vi "Test Save Unicode Paths.vi"(8 "error in (no error)":errorcluster) -> (0 "error out":errorcluster, 3 "Pass?":bool)   [LabVIEW 2020]
uses:
  <vilib>/picture/picture.llb/imagedata.ctl
  G-Image/Image IO/Polymorphic VIs/Save BMP Image (UTF-8 Path).vi
  G-Image/Image IO/Polymorphic VIs/Save GIF Image (UTF-8 Path).vi
  G-Image/Image IO/Polymorphic VIs/Save JPG Image (UTF-8 Path).vi
  G-Image/Image IO/Polymorphic VIs/Save PNG Image (UTF-8 Path).vi
  G-Image/Image IO/Polymorphic VIs/Save QOI Image (UTF-8 Path).vi
  G-Image/Image IO/Polymorphic VIs/Save TGA Image (UTF-8 Path).vi
  G-Image/Image IO/Polymorphic VIs/Load Image (UTF-8 Path).vi
  G-Image/G-Image.lvlib
panel:
  out "Array":cluster{string, "new picture":picture}[](array[cluster])
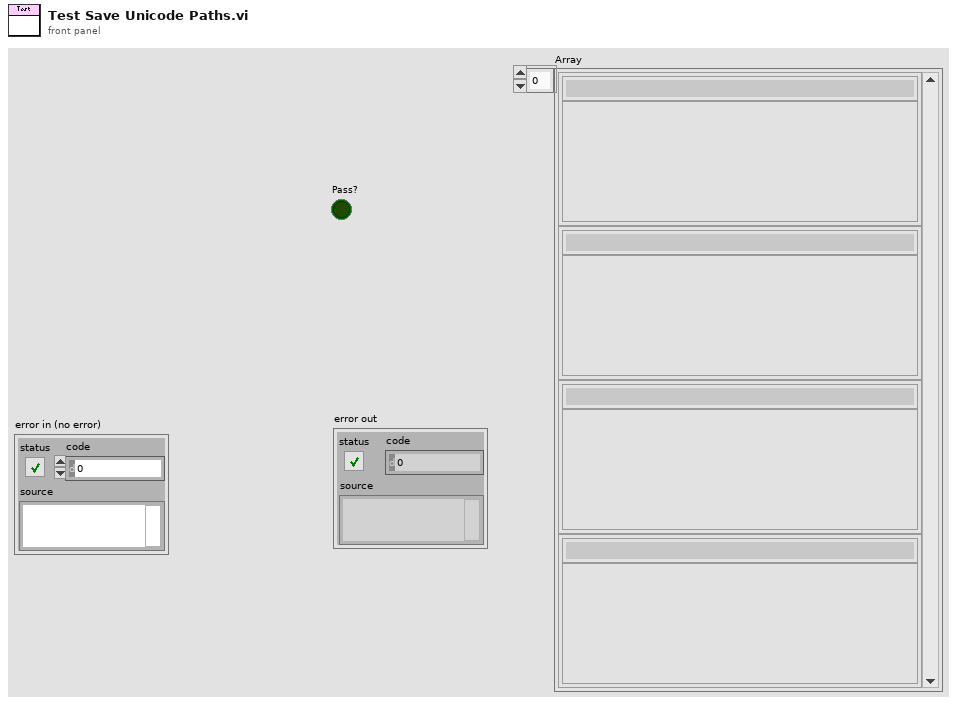
[diagram p1: front panel]
types:
  T1 = typedef "imagedata.ctl" = cluster{"image type":i32, "image depth":i32, "image":u8[], "mask":u8[], "colors":u32[], "Rectangle":cluster{"left":i16, "top":i16, "right":i16, "bottom":i16}}
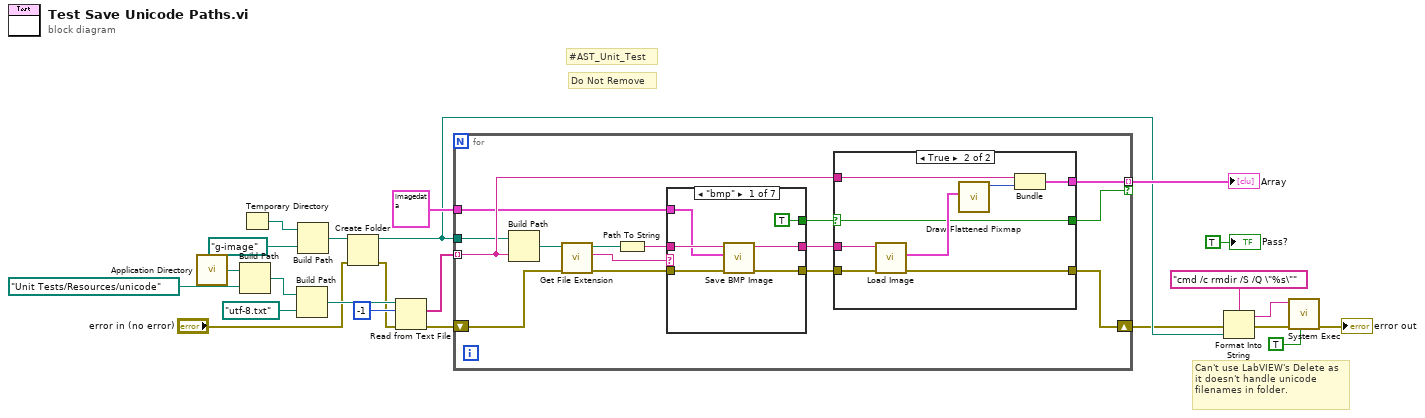
[diagram p0: block diagram]
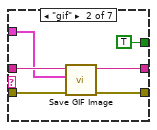
[diagram p3: hidden frame]
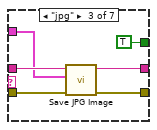
[diagram p4: hidden frame]
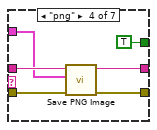
[diagram p5: hidden frame]
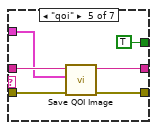
[diagram p6: hidden frame]
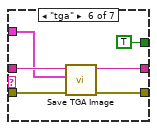
[diagram p7: hidden frame]
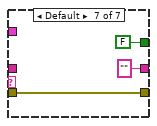
[diagram p8: hidden frame]
diagram:
  # "Can't use LabVIEW's Delete as it doesn't handle unicode filenames in folder."
  # "Do Not Remove"
  # "#AST_Unit_Test"
  n1 = call <vilib>:"Application Directory.vi"() -> ("Application Directory"=w22:path)
  n2 = Build Path(base path=w22, name or relative path=path "Unit Tests/Resources/unicode" ("Path")) -> (appended path=w16:path)
  n3 = Temporary Directory() -> (w14:path)
  n4 = Build Path(base path=w16, name or relative path=path "utf-8.txt") -> (appended path=w19:path)
  n5 = Build Path(base path=w14, name or relative path=path "g-image") -> (appended path=w13:path)
  n6 = Create Folder(path (use dialog)=w13, error in="error in (no error)") -> (created path=w8:path, error out=w1:errorcluster)  [unwired: 1 in, 1 out]
  n7 = Read from Text File(file (use dialog)=w19, count=-1 ("count (1)"), error in=w1) -> (text=w17:string[], error out=w15:errorcluster)  [unwired: 1 in, 2 out]
  n8 = for {
    shift-right: [w26] -> w7
    shift-left: w15 -> [w36]
    tunnel: [w38] -> w23 mode=indexing if=w24
    tunnel: w17 -> [w31] mode=indexing
    tunnel: w8 -> [w30]
    tunnel: T1 {"image type"=0, "image depth"=24, "image"=array[115500 elements], "mask"=[], "colors"=[], "Rectangle"={"left"=0, "top"=0, "right"=350, "bottom"=110}} ("Image") -> [w29]
    n9 = Build Path(base path=w30, name or relative path=w31) -> (appended path=w35:path)
    n10 = call <vilib>:"Get File Extension.vi"("error in (no error)"=w36, "file"=w35) -> ("error out"=w32:errorcluster, "lowercase file extension"=w33:string, "dup file"=w34:path)  [unwired: 5 in, 2 out]
    n11 = Path To String(path=w34) -> (string=w37:string)
    n12 = case shown="\"bmp\"" w33 {
      tunnel: w37 -> [w54 w60 w66 w72 w78 w84 _]
      tunnel: w32 -> [w53 w59 w65 w71 w77 w83 w86]
      tunnel: [w52 w58 w64 w70 w76 w82 w86] -> w27
      tunnel: w29 -> [w51 w57 w63 w69 w75 w81 _]
      tunnel: [w50 w56 w62 w68 w74 w80 "" ("Path Out")] -> w28
      tunnel: [TRUE TRUE TRUE TRUE TRUE TRUE FALSE] -> w25
      frame "bmp" {
        n13 = call-poly "Save BMP Image.vi"("error in (no error)"=w53, "Image"=w51, "Path In"=w54) -> ("error out"=w52:errorcluster, "Path Out"=w50:string)  [unwired: 7 in]
      }
      frame "gif" {
        n14 = call-poly "Save GIF Image.vi"("error in (no error)"=w59, "Image"=w57, "Path In"=w60) -> ("error out"=w58:errorcluster, "Path Out"=w56:string)  [unwired: 7 in]
      }
      frame "jpg" {
        n15 = call-poly "Save JPG Image.vi"("error in (no error)"=w65, "Image"=w63, "Path In"=w66) -> ("error out"=w64:errorcluster, "Path Out"=w62:string)  [unwired: 7 in]
      }
      frame "png" {
        n16 = call-poly "Save PNG Image.vi"("error in (no error)"=w71, "Image"=w69, "Path In"=w72) -> ("error out"=w70:errorcluster, "Path Out"=w68:string)  [unwired: 7 in]
      }
      frame "qoi" {
        n17 = call-poly "Save QOI Image.vi"("error in (no error)"=w77, "Image"=w75, "Path In"=w78) -> ("error out"=w76:errorcluster, "Path Out"=w74:string)  [unwired: 7 in]
      }
      frame "tga" {
        n18 = call-poly "Save TGA Image.vi"("error in (no error)"=w83, "Image"=w81, "Path In"=w84) -> ("error out"=w82:errorcluster, "Path Out"=w80:string)  [unwired: 7 in]
      }
      frame Default {
      }
    }
    n19 = case shown="True" w25 {
      selector: w25 -> [w40 w41]
      tunnel: [_ w48] -> w38
      tunnel: w31 -> [_ w47]
      tunnel: w28 -> [_ w44]
      tunnel: w27 -> [w39 w43]
      tunnel: [w39 w42] -> w26
      tunnel: [w40 w41] -> w24
      frame False {
      }
      frame True {
        n20 = call-poly "Load Image.vi"("error in (no error)"=w43, "Path In"=w44) -> ("error out"=w42:errorcluster, "Image"=w45:T1)  [unwired: 7 in, 1 out]
        n21 = call <vilib>:"Draw Flattened Pixmap.vi"("image data"=w45) -> ("new picture"=w46:picture)  [unwired: 8 in]
        n22 = Bundle(w47, "new picture"=w46) -> (w48:cluster{string, "new picture":picture})  [unwired: 1 in]
      }
    }
  }
  "Array" <- w23
  n23 = Format Into String(format string="cmd /c rmdir /S /Q \"%s\"", error in=w7, w8) -> (resulting string=w5:string, error out=w6:errorcluster)  [unwired: 1 in]
  n24 = call <vilib>:"System Exec.vi"("run minimized? (F)"=TRUE, "error in (no error)"=w6, "command line"=w5) -> ("error out"=→"error out":errorcluster)  [unwired: 5 in, 3 out]
  "Pass?" <- TRUE ("Pass?")
